vi "Get Specific Channel Resources.vi"(10 "Channel":string, 11 "Resource Name":refnum<k15>) -> (3 "Resource Name":refnum<k15>)   [LabVIEW 2023]
panel:
  out "String":string
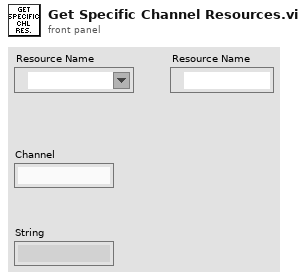
[diagram p1: front panel]
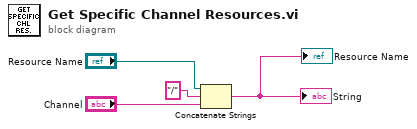
[diagram p0: block diagram]
diagram:
  n1 = Concatenate Strings("Resource Name", "/" ("string"), "Channel") -> (→"String" →"Resource Name":string)
